vi "SCCAPI Provider Supports Functionality.vi"(8 "error in (no error)":errorcluster, 10 "functionality":T1) -> (0 "error out":errorcluster, 2 "provider supports?":bool)   [LabVIEW 2017, in "NI_SCC.lvlib"]
uses:
  <vilib>/SourceControl/sccapi/NI_SCC.lvlib
  <vilib>/SourceControl/sccapi/SCCAPI SCC Provider Functionality.ctl
  <vilib>/SourceControl/sccapi/SCCAPI SCC Operations.ctl
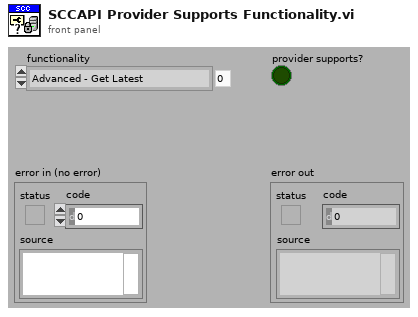
[diagram p1: front panel]
types:
  T1 = typedef "NI_SCC.lvlib/SCCAPI SCC Provider Functionality.ctl" = enum16{"Advanced - Get Latest", "Advanced - CheckOut", "Advanced - CheckIn", "Advanced - UndoCheckOut", "Advanced - Add", "Advanced - Remove", "Advanced - FileCompare", "Advanced - FileHistory", "Advanced - FileProperties", "Advanced - ConfigOptions", "Run SCC", "Configure Project", "Comment on CheckOut", "Comment on CheckIn", "Comment on Add", "Comment on Remove", "Keep Checked Out", "Get File Copy", "Multifile History"}
  T2 = typedef "NI_SCC.lvlib/SCCAPI SCC Operations.ctl" = enum16{"Add", "Check In", "Check Out", "Close Project", "Compare Files", "Compare VIs", "Configure Project", "File History", "File Properties", "File Status", "Find All Providers", "Get Advanced Command Options", "Get File Copy", "Get Latest Version", "Get Project Name", "Get StaticVI Path", "Initialize", "Not A Source Control Reference", "Open Project", "Provider Supports Functionality", "Remove", "Run Provider", "Undo Check Out", "Uninitialize", "Is File In Local Path"}
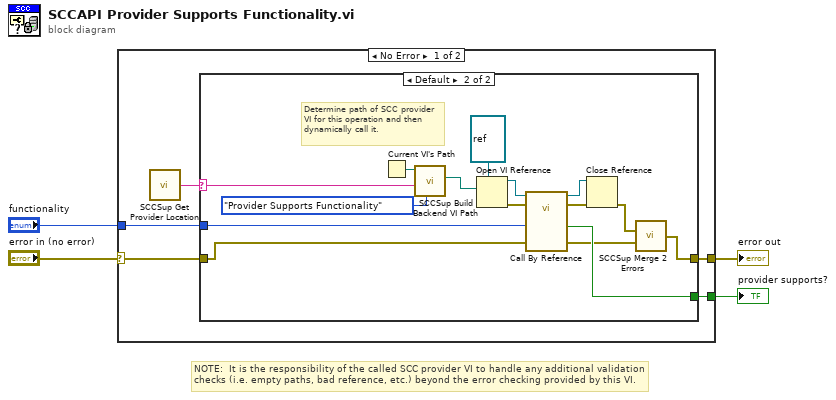
[diagram p0: block diagram]
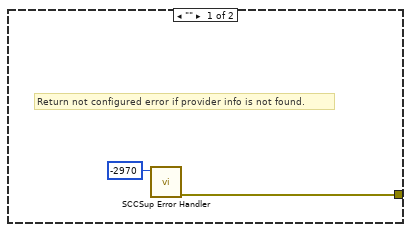
[diagram p2: hidden frame]
diagram:
  # "NOTE:  It is the responsibility of the called SCC provider VI to handle any additional validation checks (i.e. empty paths, bad reference, etc.) beyond the error checking provided by this VI."
  n1 = case shown="No Error" "error in (no error)" {
    selector: "error in (no error)" -> [w5 w27]
    tunnel: [w9 w27] -> w3
    tunnel: [w8 _] -> w2
    tunnel: "functionality" -> [w7 _]
    frame No Error {
      n2 = call <vilib>:"SCCSup Get Provider Location.vi"() -> ("provider location"=w6:string)  [unwired: 6 in]
      n3 = case shown="Default" w6 {
        selector: w6 -> [_ w13]
        tunnel: [w10 w26] -> w9
        tunnel: [_ w20] -> w8
        tunnel: w7 -> [_ w19]
        tunnel: w5 -> [_ w12]
        frame "" {
          # "Return not configured error if provider info is not found."
          n4 = call <vilib>:"SCCSup Error Handler.vi"("scc error code"=-2970 ("code")) -> ("error out"=w10:errorcluster)  [unwired: 10 in]
        }
        frame Default {
          # "Determine path of SCC provider VI for this operation and then dynamically call it."
          n5 = Current VI's Path() -> (path=w14:path)
          n6 = call <vilib>:"SCCSup Build Backend VI Path.vi"("scc operation"=SCCAPI_SCC_Operations."Provider Supports Functionality", "provider location"=w13, "caller path"=w14) -> ("scc backend VI path"=w16:path)  [unwired: 8 in]
          n7 = Open VI Reference(type specifier VI Refnum (for type only)=refnum<vi> refnum, vi path=w16) -> (vi reference=w24:refnum<vi>, error out=w23:errorcluster)  [unwired: 4 in]
          n8 = call-by-ref "?"(reference=w24, error in=w23, "error in (no error)"=w12, "functionality"=w19) -> (reference out=w22:refnum<vi>, error out=w21:errorcluster, 0:"error out"=w17:errorcluster, "provider supports?"=w20:bool)  [unwired: 8 in]
          n9 = Close Reference(reference=w22, error in (no error)=w21) -> (error out=w18:errorcluster)
          n10 = call <vilib>:"SCCSup Merge 2 Errors.vi"("Error IO 1"=w18, "Error IO 2"=w17) -> ("Error IO out"=w26:errorcluster)  [unwired: 13 in]
        }
      }
    }
    frame Error {
    }
  }
  "error out" <- w3
  "provider supports?" <- w2
